vi "z010查询壳体返工数量.vi"(8 "error in (no error)":errorcluster, 11 "转向器总成ID":string="4BSHL0714E3DE") -> (0 "error out":errorcluster, 2 "Rows Fetched":i32, 3 "无重号":bool)   [LabVIEW 2013]
uses:
  <vilib>/Utility/error.llb/whitespace.ctl
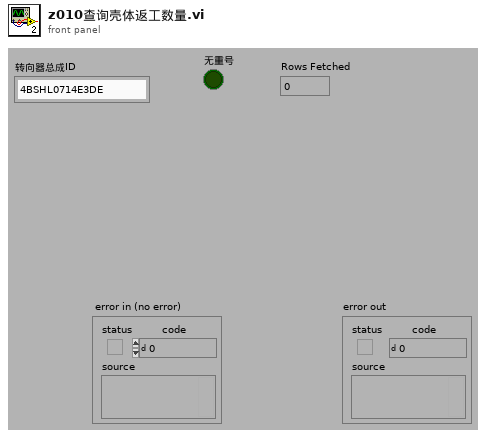
[diagram p1: front panel]
types:
  T1 = typedef "whitespace.ctl" = u16
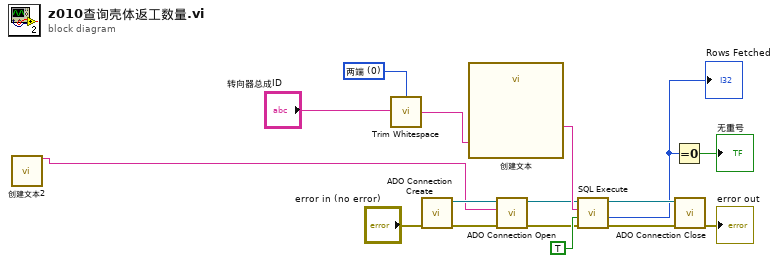
[diagram p0: block diagram]
diagram:
  w2 = T1 0 items=["两端", "字符串首端", "字符串末端"] ("location (both)")
  n1 = call "创建文本2"() -> ("Result"=w4:string)  [unwired: 14 in, 1 out]
  n2 = call <vilib>:"Trim Whitespace.vi"("string"="转向器总成ID", "location (both)"=w2) -> ("trimmed string"=w1:string)
  n3 = call "ADO Connection Create.vi"("error in (no error)"="error in (no error)") -> ("error out"=w15:errorcluster, "ADODB._Connection Out"=w16:refnum<k7>)  [unwired: 9 out]
  n4 = call "创建文本"("产品ID"=w1) -> ("Result"=w11:string)  [unwired: 13 in, 1 out]
  n5 = call "ADO Connection Open.vi"("error in (no error)"=w15, "ConnectionString"=w4, "ADODB._Connection In"=w16) -> ("error out"=w9:errorcluster, "ADODB._Connection Out"=w10:refnum<k7>)  [unwired: 7 out]
  n6 = call "SQL Execute.vi"("error in (no error)"=w9, "Return Data (T)"=TRUE, "Command Text"=w11, "ADODB._Connection In"=w10) -> ("error out"=w7:errorcluster, "Rows Fetched"=w6:i32, "ADODB._Connection Out"=w8:refnum<k7>)  [unwired: 4 in, 1 out]
  "Rows Fetched" <- w6
  n7 = Equal To 0?(x=w6) -> (x = 0?=→"无重号":bool)
  n8 = call "ADO Connection Close.vi"("error in (no error)"=w7, "ADODB._Connection In"=w8) -> ("error out"=→"error out":errorcluster)  [unwired: 9 out]
